vi "Initialize SharedRsc Attribute.vi"() -> (3 "Attribute.SharedResource":refnum<class "Attribute.SharedResource.lvclass">)   [LabVIEW 2021, in "smo.lvlib" / "Attribute.SharedResource.lvclass"]
uses:
  Attribute.SharedResource.lvclass
  C:/Repositories/SMO/src/Support/Attribute/Attribute.lvclass
  Definitions/def.SMO/Scope -- Enum.ctl
  Attribute/Attribute.lvclass/Attribute.ctl
  Attribute.SharedResource.lvclass/Attribute.SharedResource.ctl
  Definitions/def.SMO/def.SMO.lvclass
  Attribute/Attribute.lvclass
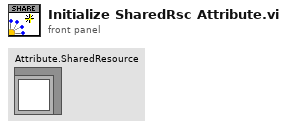
[diagram p1: front panel]
types:
  T1 = typedef "smo.lvlib/def.SMO.lvclass/Scope -- Enum.ctl" = enum16{"Public", "Protected", "Private"}
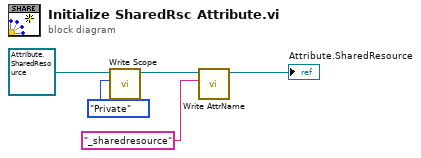
[diagram p0: block diagram]
diagram:
  n1 = call "Write Scope.vi"("Scope"=Scope_--_Enum."Private", "Attribute in"=refnum<class "Attribute.SharedResource.lvclass"> refnum ("Attribute.Owner in")) -> ("Attribute out"=w4:refnum<class "Attribute.SharedResource.lvclass">)  [unwired: 9 in]
  n2 = call "Write AttrName.vi"("Attribute Name"="_sharedresource", "Attribute in"=w4) -> ("Attribute in"=→"Attribute.SharedResource":refnum<class "Attribute.SharedResource.lvclass">)  [unwired: 9 in]
